vi "SetMixerFrequency.vi"(8 "error in (no error)":errorcluster, 10 "Mixer freq [MHz]":dbl, 11 "Scope5785_six_channel":refnum<class "Scope5782_six_channel.lvclass">) -> (0 "error out":errorcluster, 3 "Scope5785_six_channel Out":refnum<class "Scope5782_six_channel.lvclass">)   [LabVIEW 2018, in "Scope5782_six_channel.lvclass"]
uses:
  Scope5782_six_channel.lvclass
  Scope5782_six_channel.lvclass/Scope5782_six_channel.ctl
  <vilib>/Utility/error.llb/Error Cluster From Error Code.vi
  <vilib>/rvi/errors/niLvFpgaAdjustHostInterfaceError.vi
  <vilib>/rvi/interface/nirviReadWriteControl/nirviReadWriteControl.xnode
  FpgaRef/FpgaRefBase/Common FPGA ref.ctl
  FpgaRef/FpgaRef5761/FpgaRef5761.lvclass
  FpgaRef/FpgaRef5782/FpgaRef5782.lvclass
  NiFpgaLv.dll
  <vilib>/rvi/interface/Simulation/niFpgaSimulationCallBeginRW.vi
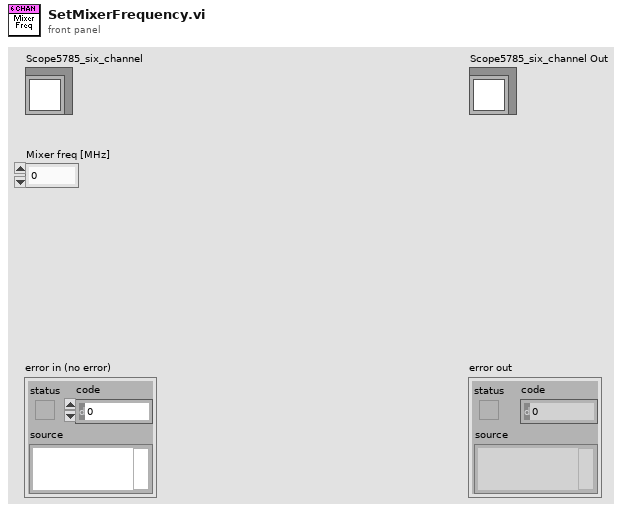
[diagram p1: front panel]
types:
  T1 = typedef "Common FPGA ref.ctl" = refnum<k20>
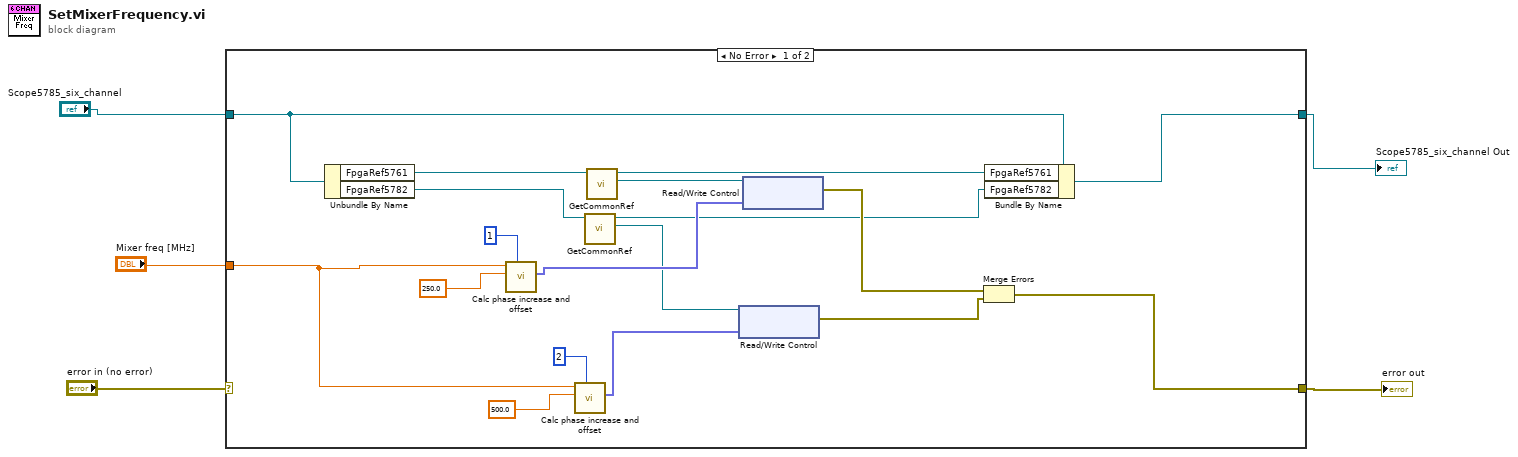
[diagram p0: block diagram]
diagram:
  n1 = case shown="No Error" "error in (no error)" {
    selector: "error in (no error)" -> [_ w24]
    tunnel: [w16 w24] -> w3
    tunnel: [w21 w23] -> w2
    tunnel: "Scope5785_six_channel" -> [w22 w23]
    tunnel: "Mixer freq [MHz]" -> [w13 _]
    frame No Error {
      n2 = Unbundle By Name(w22) -> ("FpgaRef5761"=w9:refnum<class "FpgaRef5761.lvclass">, "FpgaRef5782"=w11:refnum<class "FpgaRef5782.lvclass">)
      n3 = call "Calc phase increase and offset.vi"("# of DDS"=1, "fclk (MHz)"=250.0 ("fclk (800MHz)"), "f_generated (MHz)"=w13) -> ("Phase out"=w18:fxp<+,64,64>[])  [unwired: 6 in, 2 out]
      n4 = call "Calc phase increase and offset.vi"("# of DDS"=2, "fclk (MHz)"=500.0 ("fclk (800MHz)"), "f_generated (MHz)"=w13) -> ("Phase out"=w8:fxp<+,64,64>[])  [unwired: 6 in, 2 out]
      n5 = call-dynamic "GetCommonRef.vi"("FpgaRef5782 In"=w11) -> ("Common ref"=w7:T1, "FpgaRef5782 Out"=w10:refnum<class "FpgaRef5782.lvclass">)  [unwired: 8 in, 1 out]
      n6 = call-dynamic "GetCommonRef.vi"("FpgaRef5761 in"=w9) -> ("Common ref"=w12:T1)  [unwired: 8 in, 2 out]
      n7 = xnode "Read/Write Control"("FPGA VI Reference In"=w7, "Phase input"=w8) -> ("error out"=w6:errorcluster)  [unwired: 1 in, 1 out]
      n8 = xnode "Read/Write Control"("FPGA VI Reference In"=w12, "Phase input"=w18) -> ("error out"=w17:errorcluster)  [unwired: 1 in, 1 out]
      n9 = Merge Errors(w17, w6) -> (w16:errorcluster)
      n10 = Bundle By Name(cluster=w22, "FpgaRef5761"=w9, "FpgaRef5782"=w10) -> (w21:refnum<class "Scope5782_six_channel.lvclass">)
    }
    frame Error {
    }
  }
  "error out" <- w3
  "Scope5785_six_channel Out" <- w2
